vi "Read Input Port.vi"(8 "error in (no error)":errorcluster {"code" format="%.0x"}, 11 "VISA resource name":refnum<visa-resource-name>) -> (0 "error out":errorcluster {"code" format="%.0x"}, 2 "Data":i32, 3 "VISA resource name out":refnum<visa-resource-name>)   [LabVIEW 2016, in "Agilent N6700 Series.lvlib"]
doc: "Reads the state of the digital control port."
uses:
  <instrlib>/Agilent N6700 Series/Agilent N6700 Series.lvlib
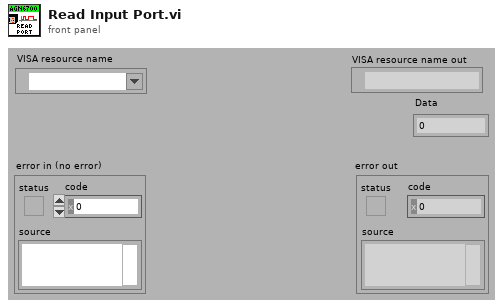
[diagram p1: front panel]
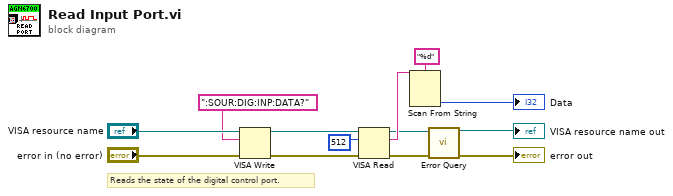
[diagram p0: block diagram]
diagram:
  # "Reads the state of the digital control port."
  n1 = VISA Write(VISA resource name="VISA resource name", write buffer=":SOUR:DIG:INP:DATA?", error in (no error)="error in (no error)") -> (VISA resource name out=w9:refnum<visa-resource-name>, error out=w8:errorcluster)  [unwired: 1 out]
  n2 = VISA Read(VISA resource name=w9, byte count=u32 512, error in (no error)=w8) -> (VISA resource name out=w2:refnum<visa-resource-name>, read buffer=w7:string, error out=w1:errorcluster)  [unwired: 1 out]
  n3 = Scan From String(format string="%d", input string=w7) -> (output 1=→"Data":i32)  [unwired: 3 in, 3 out]
  n4 = call <instrlib>:"Error Query.vi"("VISA resource name"=w2, "error in (no error)"=w1) -> ("VISA resource name out"=→"VISA resource name out":refnum<visa-resource-name>, "error out"=→"error out":errorcluster)  [unwired: 10 in, 2 out]
